vi "customized sensor for height measurementFINAL.vi"() -> ()   [LabVIEW 2022 SP3]
uses:
  <vilib>/DAQmx/create/channels.llb/DAQmx Create Channel (AI-Voltage-Basic).vi
  <vilib>/DAQmx/miscellaneous.llb/DAQmx Fill In Error Info.vi
  <vilib>/DAQmx/read.llb/DAQmx Read (Analog DBL 1Chan 1Samp).vi
panel:
  out "Height of the plant (cm)":dbl
  in  "VISA Refnum in 5":refnum<visa-resource-name>
  in  "VISA Refnum in 4":refnum<visa-resource-name>
  in  "VISA Refnum in 3":refnum<visa-resource-name>
  in  "Numeric":dbl
  out "sensor reading":dbl format="%0.2f"
  in  "physical channels":tag
  in  "stop":bool
  in  "VISA Refnum in to turn off Light":refnum<visa-resource-name>
  in  "VISA Refnum to turn on Light":refnum<visa-resource-name>
  in  "Switch":bool
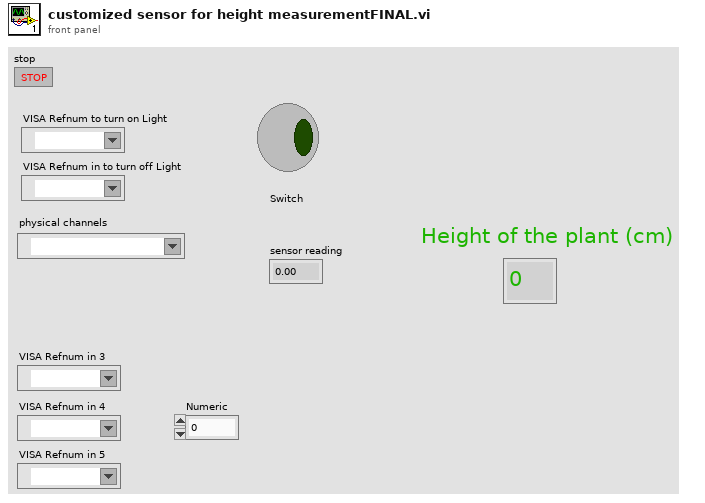
[diagram p1: front panel]
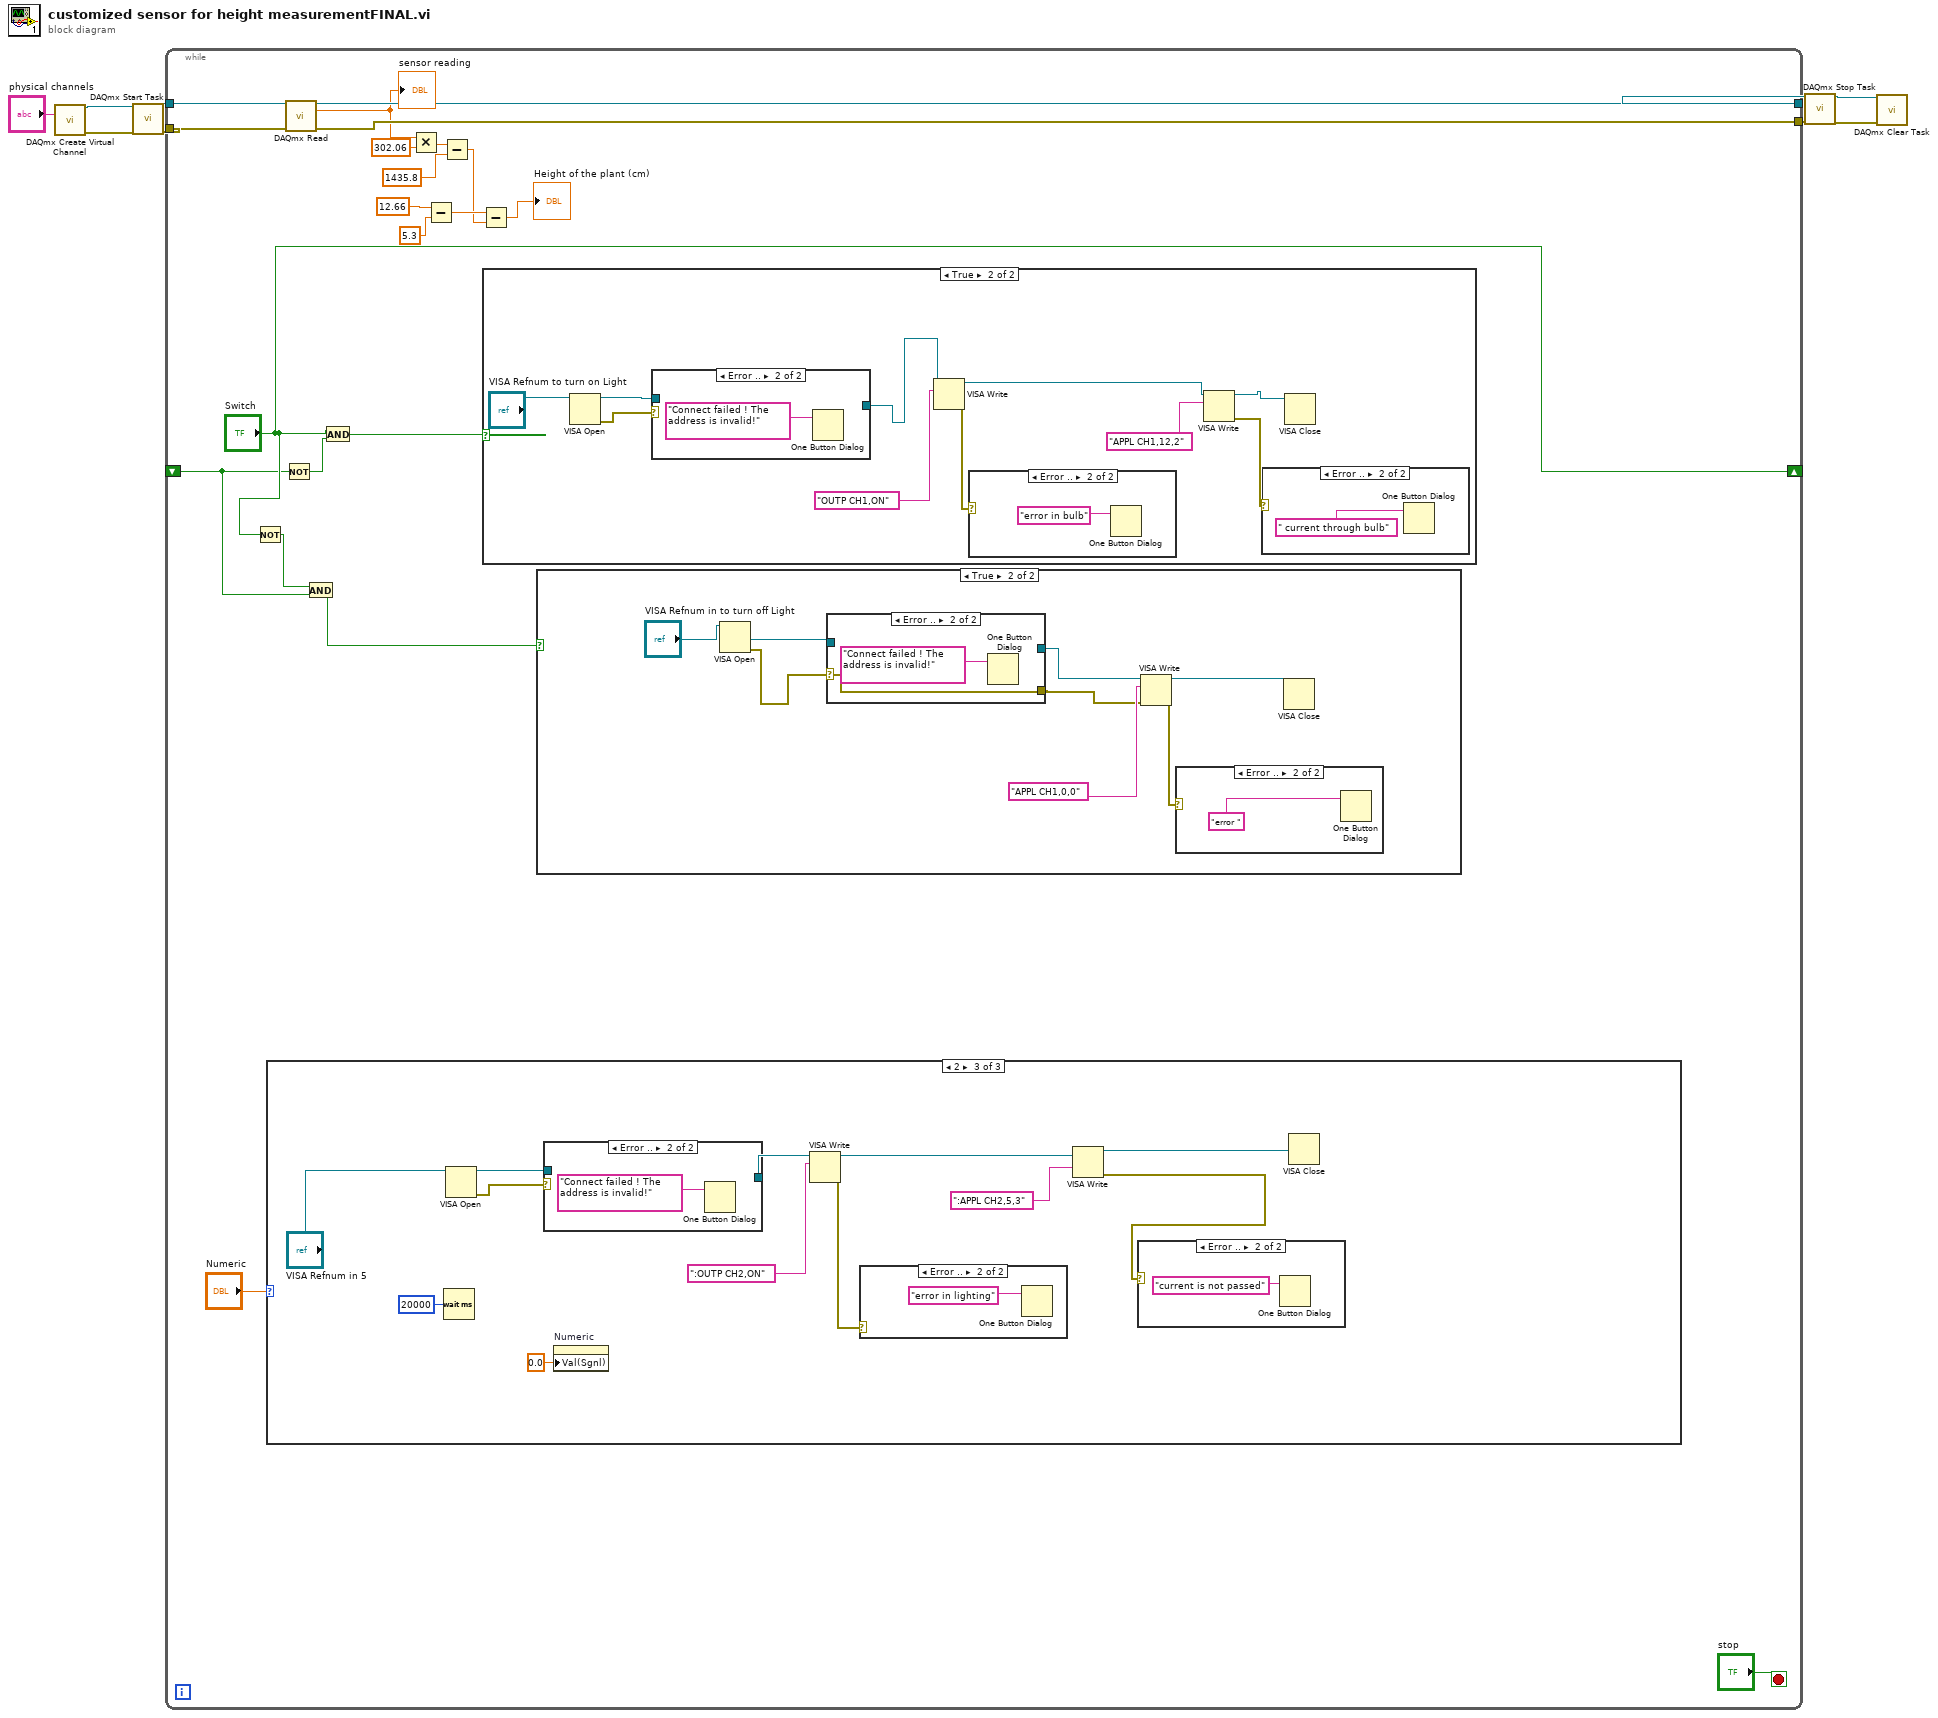
[diagram p0: block diagram]
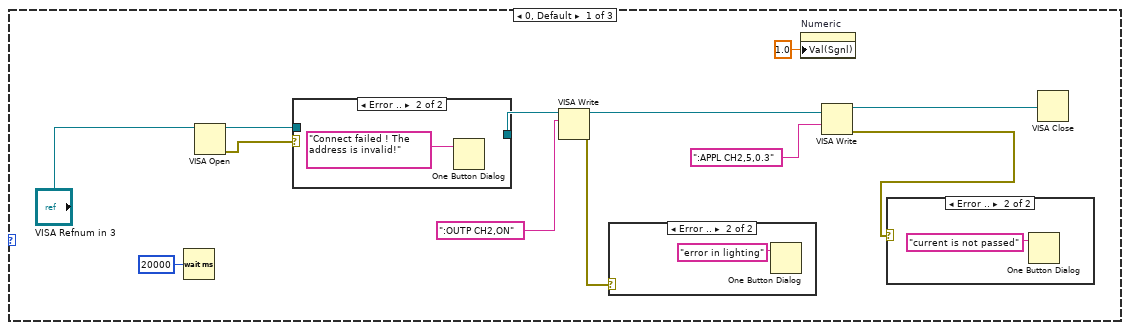
[diagram p2: hidden frame]
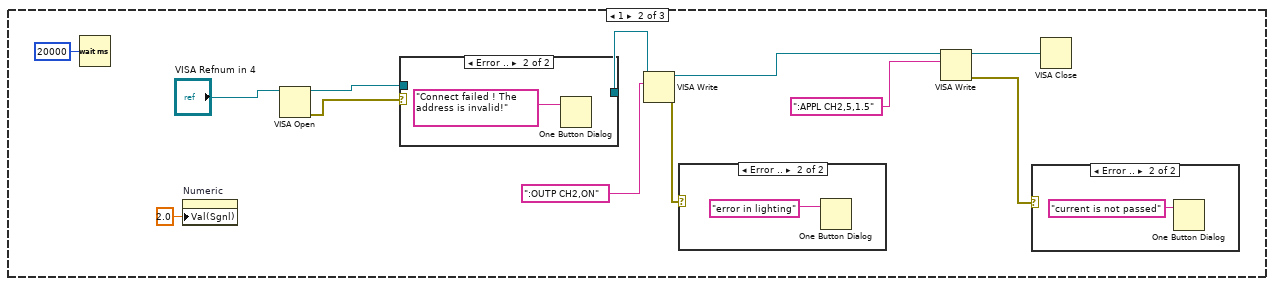
[diagram p6: hidden frame]
diagram:
  n1 = call-poly <vilib>:"DAQmx Create Virtual Channel.vi"("physical channels"="physical channels") -> ("task out"=w3:refnum<k21>, "error out"=w2:errorcluster)  [unwired: 13 in]
  n2 = call <vilib>:"DAQmx Start Task.vi"("task/channels in"=w3, "error in"=w2) -> ("task out"=w5:refnum<k21>, "error out"=w4:errorcluster)  [unwired: 12 in]
  n3 = while {
    shift-right: ["Switch"] -> _
    shift-left: _ -> [w26]
    tunnel: [w23] -> w7
    tunnel: [w22] -> w6
    tunnel: w5 -> [w21]
    tunnel: w4 -> [w20]
    stop <- "stop" stop-if-true
    n4 = Not(x="Switch") -> (.not. x?=w27:bool)
    n5 = case shown="2" "Numeric" {
      frame 0, Default {
        n6 = Wait (ms)(milliseconds to wait=u32 20000) -> ()  [unwired: 1 out]
        n7 = VISA Open(VISA resource name="VISA Refnum in 3") -> (VISA resource name=w39:refnum<visa-resource-name>, error out=w38:errorcluster)  [unwired: 4 in]
        n8 = case shown="Error .." w38 {
          tunnel: w39 -> [w45 _]
          tunnel: [w45 _] -> w36
          frame No Error {
          }
          frame Error {
            n9 = One Button Dialog(message="Connect failed ! The address is invalid!") -> ()  [unwired: 1 in, 1 out]
          }
        }
        n10 = VISA Write(VISA resource name=w36, write buffer=":OUTP CH2,ON") -> (VISA resource name out=w33:refnum<visa-resource-name>, error out=w34:errorcluster)  [unwired: 1 in, 1 out]
        n11 = case shown="Error .." w34 {
          frame No Error {
          }
          frame Error {
            n12 = One Button Dialog(message="error in lighting") -> ()  [unwired: 1 in, 1 out]
          }
        }
        n13 = property on="Numeric" class="DigNum (strict)"("Val(Sgnl)"=1.0 ("Value (Signaling)")) -> ()  [unwired: 2 in, 2 out]
        n14 = VISA Write(VISA resource name=w33, write buffer=":APPL CH2,5,0.3") -> (VISA resource name out=w40:refnum<visa-resource-name>, error out=w32:errorcluster)  [unwired: 1 in, 1 out]
        n15 = case shown="Error .." w32 {
          frame No Error {
          }
          frame Error {
            n16 = One Button Dialog(message="current is not passed") -> ()  [unwired: 1 in, 1 out]
          }
        }
        n17 = VISA Close(VISA resource name=w40) -> ()  [unwired: 1 in, 1 out]
      }
      frame 1 {
        n18 = Wait (ms)(milliseconds to wait=u32 20000) -> ()  [unwired: 1 out]
        n19 = property on="Numeric" class="DigNum (strict)"("Val(Sgnl)"=2.0 ("Value (Signaling)")) -> ()  [unwired: 2 in, 2 out]
        n20 = VISA Open(VISA resource name="VISA Refnum in 4") -> (VISA resource name=w56:refnum<visa-resource-name>, error out=w55:errorcluster)  [unwired: 4 in]
        n21 = case shown="Error .." w55 {
          tunnel: w56 -> [w61 _]
          tunnel: [w61 _] -> w54
          frame No Error {
          }
          frame Error {
            n22 = One Button Dialog(message="Connect failed ! The address is invalid!") -> ()  [unwired: 1 in, 1 out]
          }
        }
        n23 = VISA Write(VISA resource name=w54, write buffer=":OUTP CH2,ON") -> (VISA resource name out=w51:refnum<visa-resource-name>, error out=w52:errorcluster)  [unwired: 1 in, 1 out]
        n24 = case shown="Error .." w52 {
          frame No Error {
          }
          frame Error {
            n25 = One Button Dialog(message="error in lighting") -> ()  [unwired: 1 in, 1 out]
          }
        }
        n26 = VISA Write(VISA resource name=w51, write buffer=":APPL CH2,5,1.5") -> (VISA resource name out=w57:refnum<visa-resource-name>, error out=w50:errorcluster)  [unwired: 1 in, 1 out]
        n27 = case shown="Error .." w50 {
          frame No Error {
          }
          frame Error {
            n28 = One Button Dialog(message="current is not passed") -> ()  [unwired: 1 in, 1 out]
          }
        }
        n29 = VISA Close(VISA resource name=w57) -> ()  [unwired: 1 in, 1 out]
      }
      frame 2 {
        n30 = Wait (ms)(milliseconds to wait=u32 20000) -> ()  [unwired: 1 out]
        n31 = VISA Open(VISA resource name="VISA Refnum in 5") -> (VISA resource name=w72:refnum<visa-resource-name>, error out=w71:errorcluster)  [unwired: 4 in]
        n32 = case shown="Error .." w71 {
          tunnel: w72 -> [w77 _]
          tunnel: [w77 _] -> w69
          frame No Error {
          }
          frame Error {
            n33 = One Button Dialog(message="Connect failed ! The address is invalid!") -> ()  [unwired: 1 in, 1 out]
          }
        }
        n34 = property on="Numeric" class="DigNum (strict)"("Val(Sgnl)"=0.0 ("Value (Signaling)")) -> ()  [unwired: 2 in, 2 out]
        n35 = VISA Write(VISA resource name=w69, write buffer=":OUTP CH2,ON") -> (VISA resource name out=w66:refnum<visa-resource-name>, error out=w67:errorcluster)  [unwired: 1 in, 1 out]
        n36 = case shown="Error .." w67 {
          frame No Error {
          }
          frame Error {
            n37 = One Button Dialog(message="error in lighting") -> ()  [unwired: 1 in, 1 out]
          }
        }
        n38 = VISA Write(VISA resource name=w66, write buffer=":APPL CH2,5,3") -> (VISA resource name out=w73:refnum<visa-resource-name>, error out=w65:errorcluster)  [unwired: 1 in, 1 out]
        n39 = case shown="Error .." w65 {
          frame No Error {
          }
          frame Error {
            n40 = One Button Dialog(message="current is not passed") -> ()  [unwired: 1 in, 1 out]
          }
        }
        n41 = VISA Close(VISA resource name=w73) -> ()  [unwired: 1 in, 1 out]
      }
    }
    n42 = Not(x=w26) -> (.not. x?=w29:bool)
    n43 = call-poly <vilib>:"DAQmx Read.vi"("task/channels in"=w21, "error in"=w20) -> ("task out"=w23:refnum<k21>, "data"=w14:dbl, "error out"=w22:errorcluster)  [unwired: 11 in]
    "sensor reading" <- w14
    n44 = And(x=w27, y=w26) -> (x .and. y?=w25:bool)
    n45 = And(x="Switch", y=w29) -> (x .and. y?=w28:bool)
    n46 = Multiply(x=w14, y=302.06) -> (x*y=w12:dbl)
    n47 = Subtract(x=12.66, y=5.3) -> (x-y=w18:dbl)
    n48 = Subtract(x=w12, y=1435.8) -> (x-y=w10:dbl)
    n49 = Subtract(x=w18, y=w10) -> (x-y=→"Height of the plant (cm)":dbl)
    n50 = case shown="True" w28 {
      frame False {
      }
      frame True {
        n51 = VISA Open(VISA resource name="VISA Refnum to turn on Light") -> (VISA resource name=w93:refnum<visa-resource-name>, error out=w94:errorcluster)  [unwired: 4 in]
        n52 = case shown="Error .." w94 {
          tunnel: w93 -> [w104 _]
          tunnel: [w104 _] -> w96
          frame No Error {
          }
          frame Error {
            n53 = One Button Dialog(message="Connect failed ! The address is invalid!") -> ()  [unwired: 1 in, 1 out]
          }
        }
        n54 = VISA Write(VISA resource name=w96, write buffer="OUTP CH1,ON") -> (VISA resource name out=w99:refnum<visa-resource-name>, error out=w98:errorcluster)  [unwired: 1 in, 1 out]
        n55 = case shown="Error .." w98 {
          frame No Error {
          }
          frame Error {
            n56 = One Button Dialog(message="error in bulb") -> ()  [unwired: 1 in, 1 out]
          }
        }
        n57 = VISA Write(VISA resource name=w99, write buffer="APPL CH1,12,2") -> (VISA resource name out=w92:refnum<visa-resource-name>, error out=w101:errorcluster)  [unwired: 1 in, 1 out]
        n58 = case shown="Error .." w101 {
          frame No Error {
          }
          frame Error {
            n59 = One Button Dialog(message=" current through bulb") -> ()  [unwired: 1 in, 1 out]
          }
        }
        n60 = VISA Close(VISA resource name=w92) -> ()  [unwired: 1 in, 1 out]
      }
    }
    n61 = case shown="True" w25 {
      frame False {
      }
      frame True {
        n62 = VISA Open(VISA resource name="VISA Refnum in to turn off Light") -> (VISA resource name=w80:refnum<visa-resource-name>, error out=w82:errorcluster)  [unwired: 4 in]
        n63 = case shown="Error .." w82 {
          selector: w82 -> [w87 w89]
          tunnel: w80 -> [w88 _]
          tunnel: [w88 _] -> w83
          tunnel: [w87 w89] -> w79
          frame No Error {
          }
          frame Error {
            n64 = One Button Dialog(message="Connect failed ! The address is invalid!") -> ()  [unwired: 1 in, 1 out]
          }
        }
        n65 = VISA Write(VISA resource name=w83, write buffer="APPL CH1,0,0", error in (no error)=w79) -> (VISA resource name out=w84:refnum<visa-resource-name>, error out=w86:errorcluster)  [unwired: 1 out]
        n66 = case shown="Error .." w86 {
          frame No Error {
          }
          frame Error {
            n67 = One Button Dialog(message="error ") -> ()  [unwired: 1 in, 1 out]
          }
        }
        n68 = VISA Close(VISA resource name=w84) -> ()  [unwired: 1 in, 1 out]
      }
    }
  }
  n69 = call <vilib>:"DAQmx Stop Task.vi"("task/channels in"=w7, "error in"=w6) -> ("task out"=w9:refnum<k21>, "error out"=w8:errorcluster)  [unwired: 12 in]
  n70 = call <vilib>:"DAQmx Clear Task.vi"("task in"=w9, "error in"=w8) -> ()  [unwired: 13 in, 1 out]
